vi "New Driver Input.vi"(8 "error in (no error)":errorcluster, 11 "Driver-Logical in":refnum<class "Driver.lvclass">) -> (0 "error out":errorcluster, 3 "Driver-Logical out":refnum<class "Driver.lvclass">)   [LabVIEW 2013, in "Logical Systems.lvlib" / "Driver.lvlib" / "Driver.lvclass"]
uses:
  Driver.lvclass
  Drive Train/Drive Train Commands/Drive By Power/Drive by Power Class/Drive by Power.lvclass
  Robot Actors/System Actor/System Actor Messages/Start Command Msg/Start Command Msg.lvclass/Start Command Msg.ctl
  <vilib>/ActorFramework/Message Enqueuer/Message Enqueuer.lvclass/Message Enqueuer.ctl
  <vilib>/ActorFramework/Message Enqueuer/Enqueue.vi
  Virtual Robot/Robot Global.vi
  <vilib>/ActorFramework/Message Priority Queue/Priority Enqueue.vi
  Robot Actors/System Actor/System Actor Messages/Start Command Msg/Start Command Msg.lvclass
  Driver.lvlib
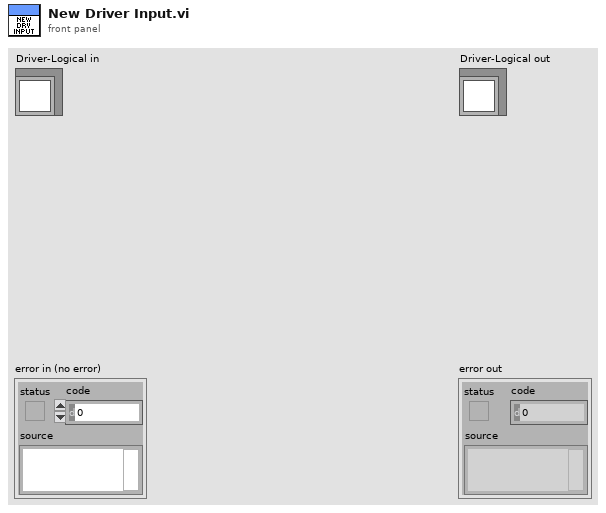
[diagram p1: front panel]
types:
  T1 = typedef "Logical Systems.lvlib/Driver.lvlib/Driver.lvclass/Driver Status.ctl" = cluster{"Current Xbox Controller":T2}
  T2 = typedef "Logical Systems.lvlib/Xbox Controller.lvlib/Xbox Controller.ctl" = cluster{"Left Joystick":T3, "Right Joystick":T3}
  T3 = typedef "Logical Systems.lvlib/Xbox Controller.lvlib/Joystick.ctl" = cluster{"Forward":dbl, "Right":dbl}
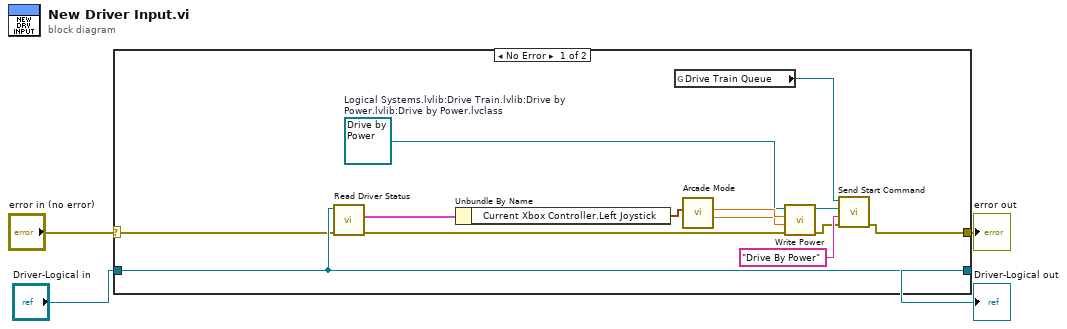
[diagram p0: block diagram]
diagram:
  n1 = case shown="No Error" "error in (no error)" {
    selector: "error in (no error)" -> [w11 w19]
    tunnel: [w5 w19] -> w3
    tunnel: [w12 w18] -> w1
    tunnel: "Driver-Logical in" -> [w12 w18]
    frame No Error {
      w13 = refnum<class "Drive by Power.lvclass"> refnum  # Logical Systems.lvlib:Drive Train.lvlib:Drive by Power.lvlib:Drive by Power.lvclass
      n2 = call-dynamic "Read Driver Status.vi"("error in (no error)"=w11, "Driver in"=w12) -> ("error out"=w10:errorcluster, "Driver Status"=w17:T1)  [unwired: 7 in, 1 out]
      n3 = Unbundle By Name(w17) -> ("Current Xbox Controller.Left Joystick"=w16:T3)
      n4 = global read "Robot Global.vi" "Drive Train Queue"() -> (w9:refnum<class "Message Enqueuer.lvclass">)
      n5 = call "Arcade Mode.vi"("Joystick In"=w16) -> ("Right Power"=w14:dbl, "Left Power"=w15:dbl)  [unwired: 9 in]
      n6 = call-dynamic "Write Power.vi"("error in (no error)"=w10, "Right Power"=w14, "Left Power"=w15, "Drive by Power in"=w13) -> ("error out"=w6:errorcluster, "Drive by Power out"=w7:refnum<class "Drive by Power.lvclass">)  [unwired: 6 in]
      n7 = call "Send Start Command.vi"("error in (no error)"=w6, "Command Name"="Drive By Power", "Robot Actors.lvlib:Command.lvlib:Command.lvclass"=w7, "Message Enqueuer"=w9) -> ("error out"=w5:errorcluster)  [unwired: 6 in, 1 out]
    }
    frame Error {
    }
  }
  "error out" <- w3
  "Driver-Logical out" <- w1
